vi "Send PUBLISH.vi"(0 "WAMP Client in":refnum<class "WAMP Client.lvclass">, 5 "Message Loop Shift Register Data (In)":T1, 7 "Publish Request Data":T4, 11 "error in (no error)":errorcluster) -> (4 "WAMP Client out":refnum<class "WAMP Client.lvclass">, 6 "Message Loop Shift Register Data (Out)":T1, 15 "error out":errorcluster)   [LabVIEW 2020, in "WAMP Client.lvclass"]
uses:
  <userlib>/lvwamp/WAMP Client/WAMP Client.lvclass
  <userlib>/lvwamp/WAMP Client/TypeDef/PUBLISH Request Data.ctl
  <userlib>/lvwamp/WAMP Client/TypeDef/PUBLISH Result.ctl
  <userlib>/lvwamp/WAMP Client/TypeDef/Message Loop Shift Reg Data.ctl
  <userlib>/lvwamp/WAMP Client/TypeDef/REGISTER Request Data.ctl
  <userlib>/lvwamp/WAMP Client/TypeDef/REGISTERED or ERROR payload.ctl
  <userlib>/lvwamp/WAMP Client/TypeDef/WAMP Error Payload.ctl
  <userlib>/lvwamp/WAMP Client/TypeDef/INVOCATION payload.ctl
  <userlib>/lvwamp/WAMP Client/TypeDef/Publish Requests Map.ctl
  <userlib>/lvwamp/WAMP Client/TypeDef/Endpoint Data.ctl
  <userlib>/lvwamp/WAMP Message Codes.ctl
  <userlib>/lvwamp/WAMP Client/WAMP Client.lvclass/WAMP Client.ctl
  <vilib>/JDP Science/JSONtext/JSONtext.lvlib
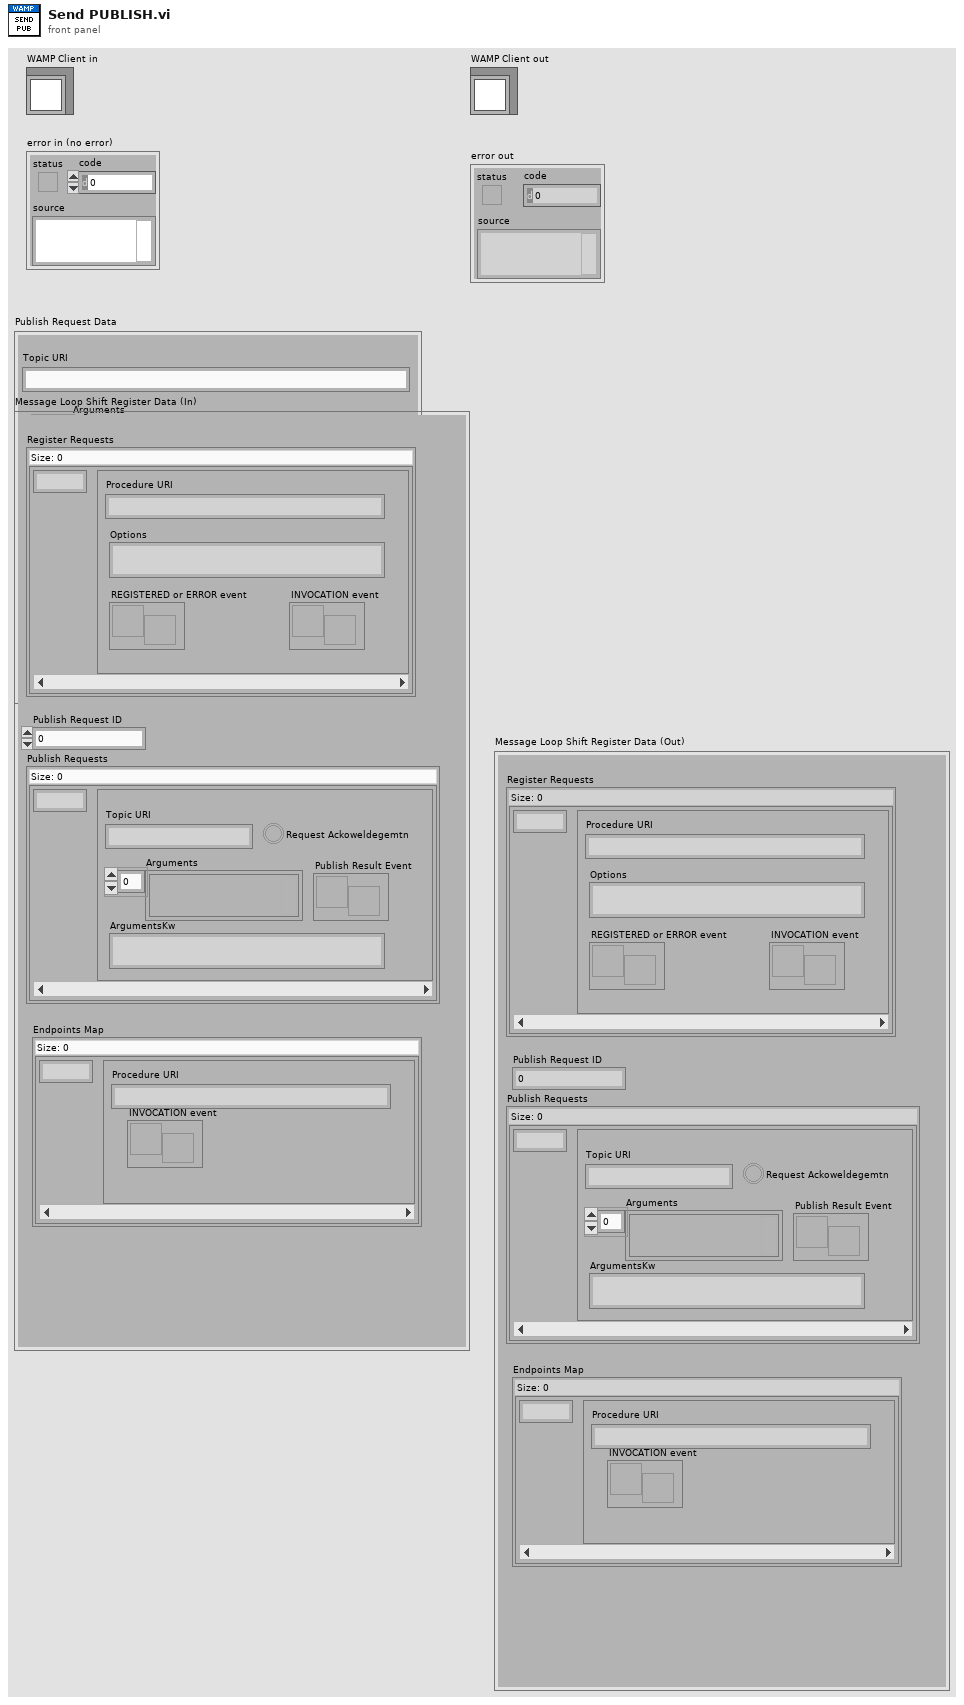
[diagram p1: front panel]
types:
  T1 = typedef "WAMP Client.lvclass/Message Loop Shift Reg Data.ctl" = cluster{"Register Requests":map{u32, T2}, "Publish Request ID":u32, "Publish Requests":T3, "Endpoints Map":map{u32, T5}}
  T2 = typedef "WAMP Client.lvclass/REGISTER Request Data.ctl" = cluster{"Procedure URI":string, "Options":string, "REGISTERED or ERROR event":refnum<user-event>, "INVOCATION event":refnum<user-event>}
  T3 = typedef "WAMP Client.lvclass/Publish Requests Map.ctl" = map{u32, T4}
  T4 = typedef "WAMP Client.lvclass/PUBLISH Request Data.ctl" = cluster{"Topic URI":string, "Arguments":variant[], "ArgumentsKw":string, "Publish Result Event":refnum<user-event>, "Request Ackoweldegemtn":bool}
  T5 = typedef "WAMP Client.lvclass/Endpoint Data.ctl" = cluster{"Procedure URI":string, "INVOCATION event":refnum<user-event>}
  T6 = typedef "WAMP Client.lvclass/WAMP Message Codes.ctl" = u16
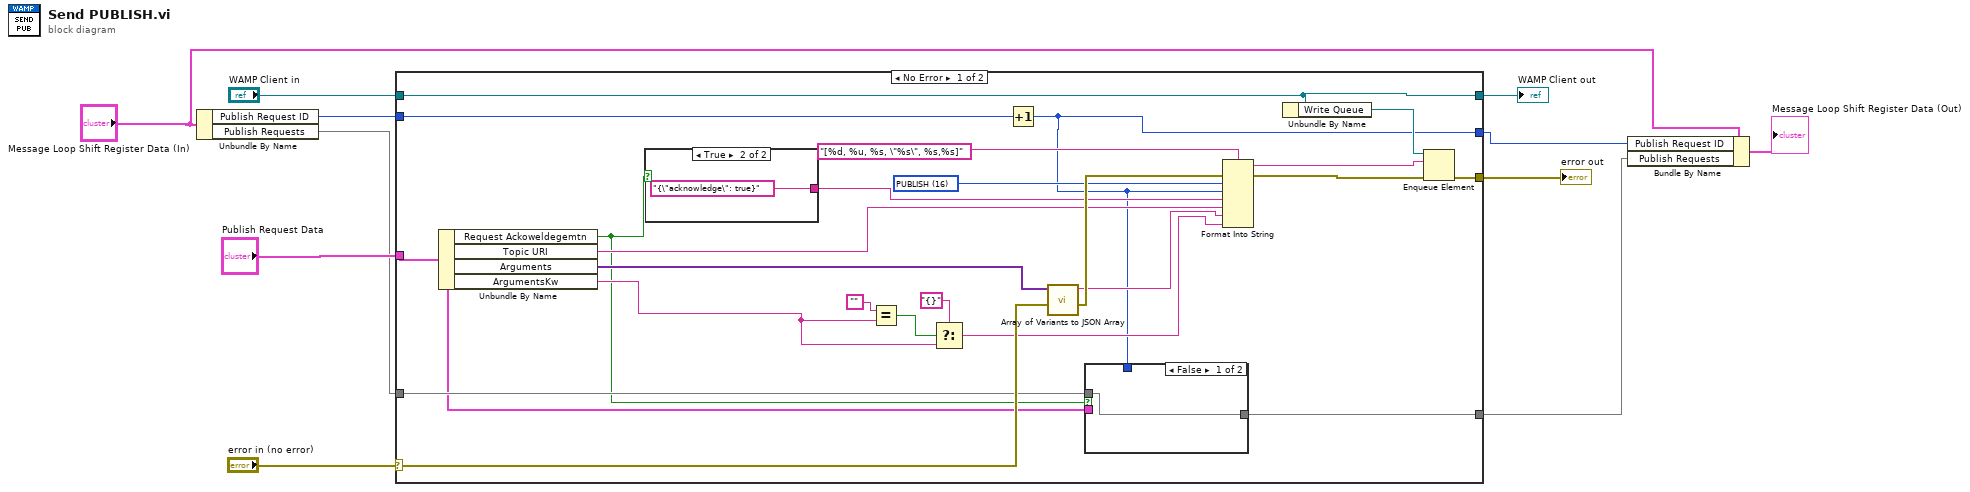
[diagram p0: block diagram]
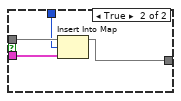
[diagram p2: hidden frame]
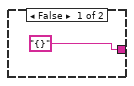
[diagram p3: hidden frame]
diagram:
  n1 = Unbundle By Name("Message Loop Shift Register Data (In)") -> ("Publish Request ID"=w5:u32, "Publish Requests"=w6:T3)
  n2 = case shown="No Error" "error in (no error)" {
    selector: "error in (no error)" -> [w27 w45]
    tunnel: [w35 w45] -> w10
    tunnel: [w24 w44] -> w8
    tunnel: "WAMP Client in" -> [w24 w44]
    tunnel: w5 -> [w25 _]
    tunnel: [w13 _] -> w3
    tunnel: "Publish Request Data" -> [w19 _]
    tunnel: w6 -> [w21 w43]
    tunnel: [w18 w43] -> w2
    frame No Error {
      w20 = T6 16 items=["HELLO"=1, "WELCOME"=2, "ABORT"=3, "GOODBYE"=6, "ERROR"=8, "PUBLISH"=16, "PUBLISHED"=17, "SUBSCRIBE"=32, "SUBSCRIBED"=33, "UNSUBSCRIBE"=34, "UNSUBSCRIBED"=35, "EVENT"=36, "CALL"=48, "RESULT"=59, "REGISTER"=64, "REGISTERED"=65, "UNREGISTER"=66, "UNREGISTERED"=67, "INVOCATION"=68, "YIELD"=70] ("Message Codes")
      n3 = Unbundle By Name(w19) -> ("Request Ackoweldegemtn"=w12:bool, "Topic URI"=w15:string, "Arguments"=w23:variant[], "ArgumentsKw"=w22:string)
      n4 = case shown="True" w12 {
        tunnel: ["{}" "{\"acknowledge\": true}"] -> w14
        frame False {
        }
        frame True {
        }
      }
      n5 = Equal?(x="", y=w22) -> (x = y?=w31:bool)
      n6 = Select(t="{}", s=w31, f=w22) -> (s? t:f=w17:string)
      n7 = Increment(x=w25) -> (x+1=w13:u32)
      n8 = call <vilib>:"Array of Variants to JSON Array.vi"("error in (no error)"=w27, "Array of Variants"=w23) -> ("error out"=w26:errorcluster, "<JSON>"=w16:string)  [unwired: 8 in]
      n9 = case shown="False" w12 {
        tunnel: w21 -> [w36 w40]
        tunnel: w19 -> [_ w39]
        tunnel: [w36 w38] -> w18
        tunnel: w13 -> [_ w37]
        frame False {
        }
        frame True {
          n10 = Insert Into Map(map in=w40, key=w37, value=w39) -> (map out=w38:T3)  [unwired: 2 out]
        }
      }
      n11 = Format Into String(format string="[%d, %u, %s, \"%s\", %s,%s]" ("element"), error in=w26, w20, w13, w14, w15, w16, w17) -> (resulting string=w33:string, error out=w32:errorcluster)  [unwired: 1 in]
      n12 = Unbundle By Name(w24) -> ("Write Queue"=w28:refnum<queue>)
      n13 = Enqueue Element(queue=w28, element=w33, error in (no error)=w32) -> (error out=w35:errorcluster)  [unwired: 1 in, 2 out]
    }
    frame Error {
    }
  }
  "error out" <- w10
  "WAMP Client out" <- w8
  n14 = Bundle By Name(cluster="Message Loop Shift Register Data (In)", "Publish Request ID"=w3, "Publish Requests"=w2) -> (→"Message Loop Shift Register Data (Out)":T1)
